vi "System-CAN-Host.vi"() -> ()   [LabVIEW 2016]
uses:
  Shared/Typedefs/System-CAN-FrameInfoArray.ctl
  Shared/Typedefs/System-CAN-FrameInfo.ctl
  <vilib>/addons/Software Calibration Management/xSCM/Controls/ID and Element.ctl
  Shared/DSI-Shared.lvlib
  <vilib>/addons/Software Calibration Management/xSCM/SCM-API.lvlib
panel:
  in  "QueueLength":u8 caption="Queue Length"
  in  "WritePeriod":u32 caption="[msec]"
  in  "Interface":u8(ring) items=["CAN 0", "CAN 1"]
  in  "BaudRate":u32 caption="[baud]"
  in  "Reset":bool
  out "WriteError":bool
  out "ReadError":bool
  in  "_WriteTable":i32(listbox) caption="Write to CAN Bus"
  in  "_ReadTable":i32(listbox) caption="Read from CAN Bus"
  in  "_Hidden":enum32{"Page 1"}(tab)
  in  "_Edit":bool
  in  "_Down":bool
  in  "_Delete":bool
  in  "_Up":bool
  in  "_Insert":bool
  out "ReadElements":i32
  out "WriteElements":i32
  in  "_Read(F)-Write(T)":bool
  in  "_Refresh":bool
  out "Read_ActIDs":sgl[](array[numeric])
  out "Read_Values":sgl[](array[numeric])
  out "Write_Values":sgl[](array[numeric])
  in  "Read_IDs":sgl[](array[numeric])
  in  "ReadFramesInfo":T1
  in  "WriteFramesInfo":T1
  in  "_CurrentFrameInfo":T2
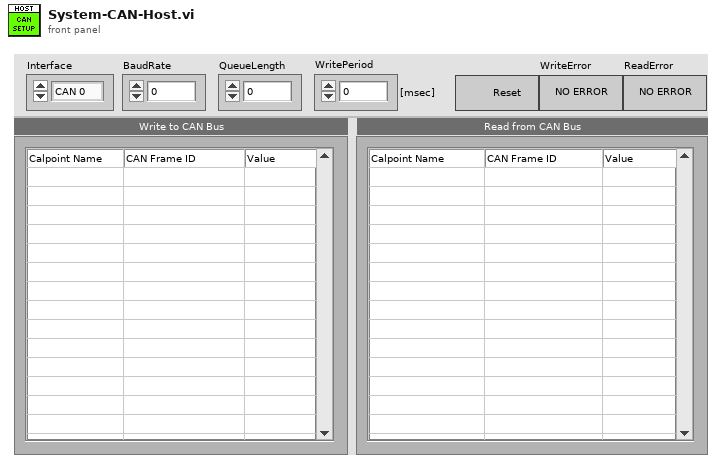
[diagram p1: front panel]
types:
  T1 = typedef "DSI-Shared.lvlib/System-CAN-FrameInfoArray.ctl" = T2[]
  T2 = typedef "DSI-Shared.lvlib/System-CAN-FrameInfo.ctl" = cluster{"Name":string, "Units":string, "Identifier":u32, "Disable":bool, "Type":u16, "Scaling Factor":sgl, "Offset":sgl, "ExtID":bool, "Min":sgl, "Max":sgl, "Number of Bits":u8, "Start Bit":u8, "Byte Order":u8, "ID":T3}
  T3 = typedef "SCM-API.lvlib/ID and Element.ctl" = cluster{"ID":u32, "Element":i32[]}
  T4 = typedef "LVBoundsTypeDef.ctl" = cluster{"Width":u32, "Height":u32}
  T5 = typedef "LVRectTypeDef.ctl" = cluster{"Left":i16, "Top":i16, "Right":i16, "Bottom":i16}
  T6 = typedef "LVRowAndColumnUnsignedTypeDef.ctl" = cluster{"Row":u32, "Column":u32}
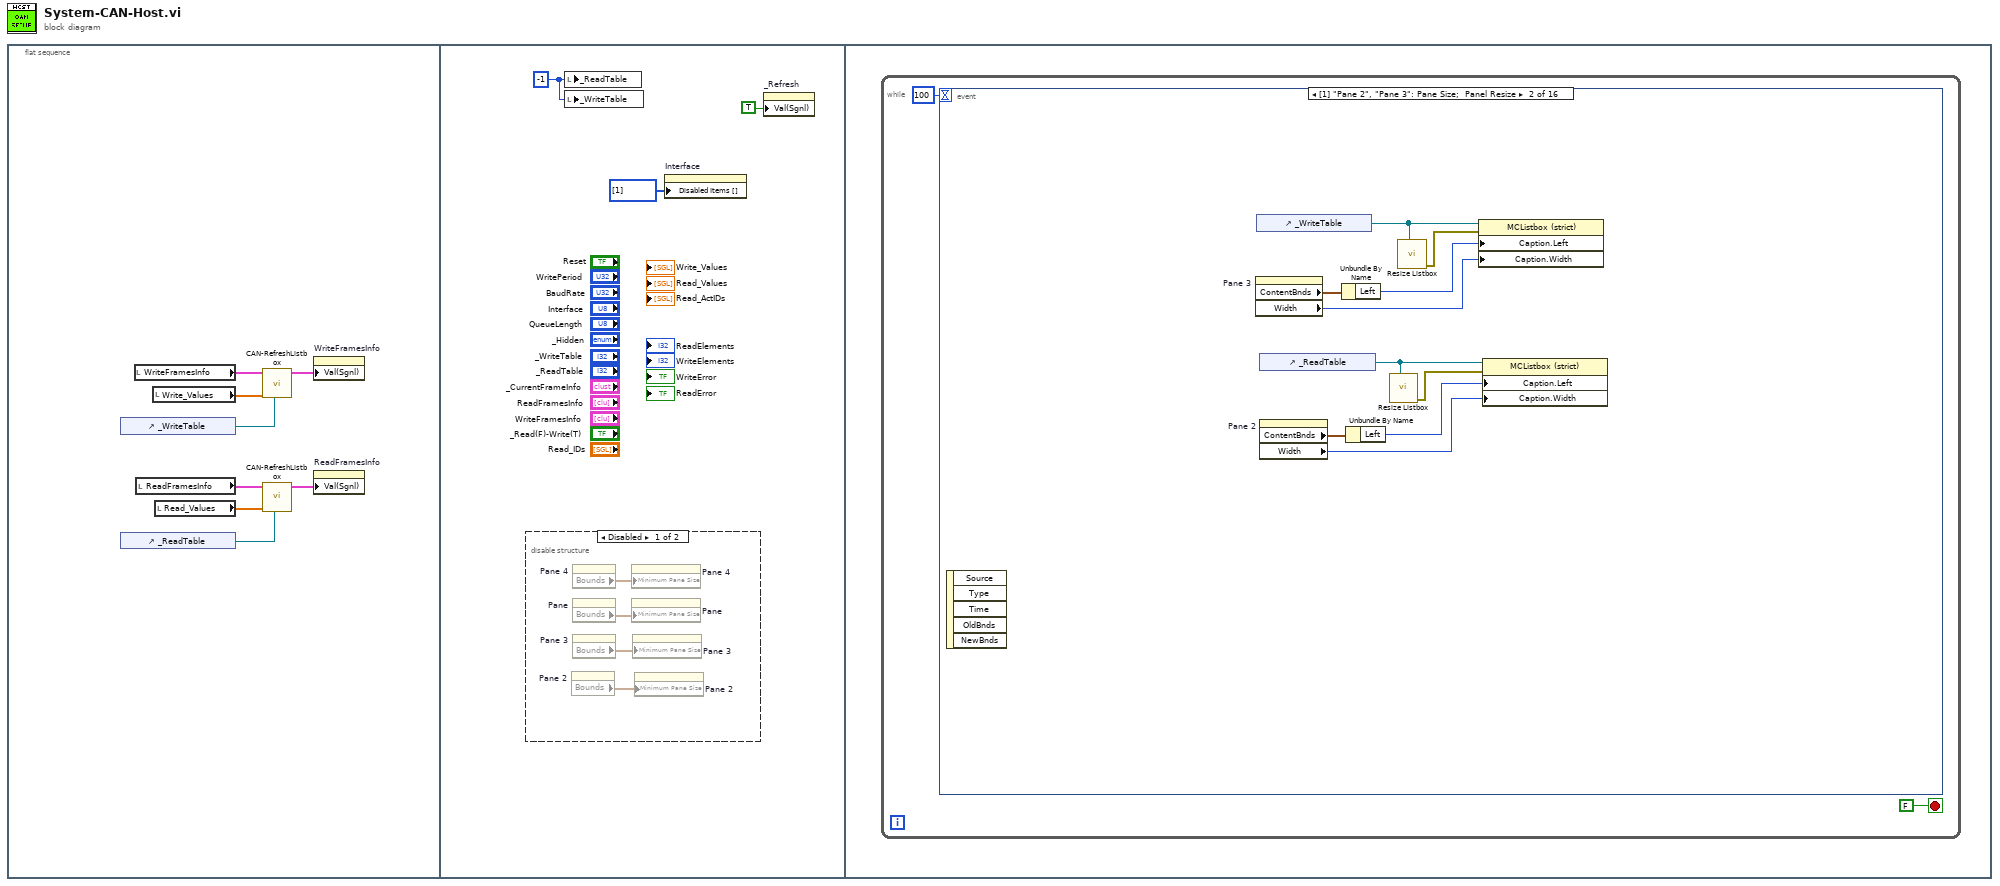
[diagram p0: block diagram]
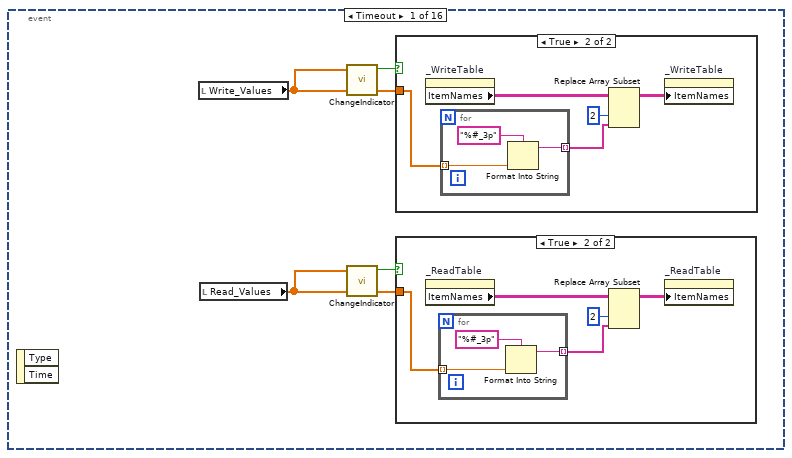
[diagram p3: hidden frame]
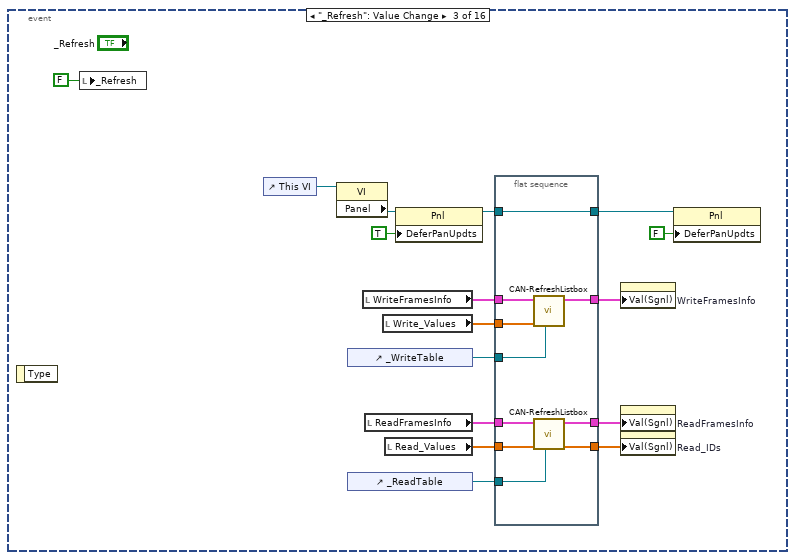
[diagram p6: hidden frame]
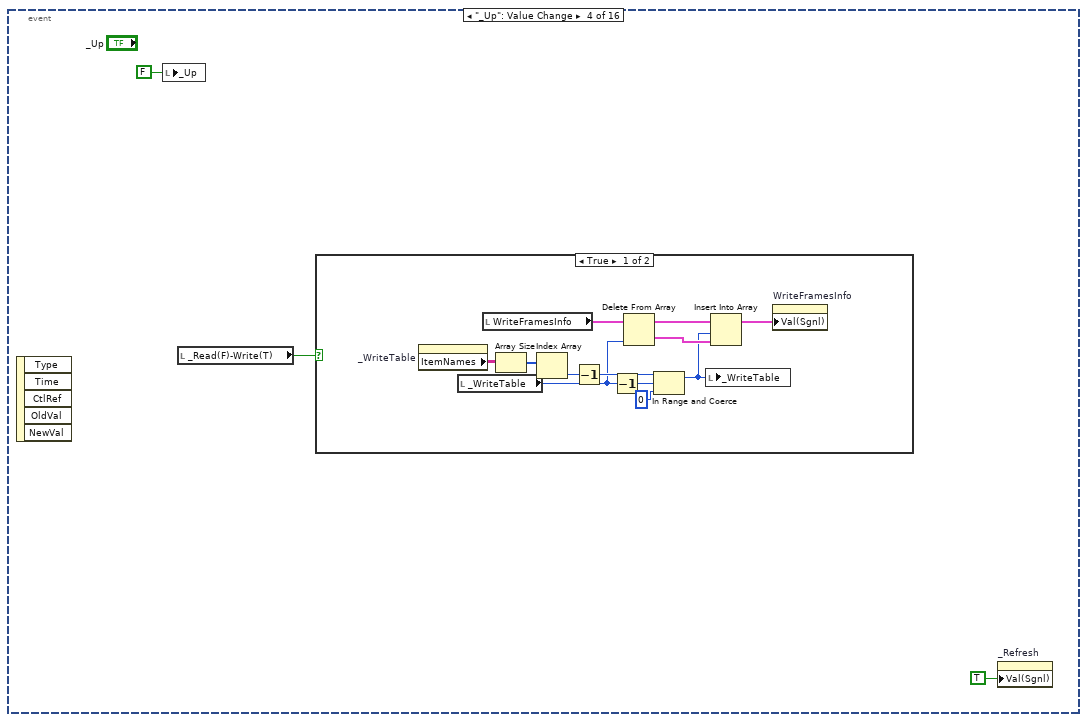
[diagram p7: hidden frame]
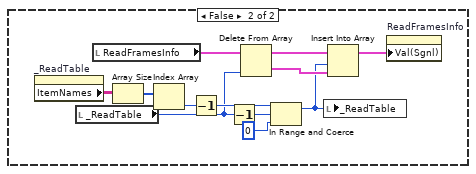
[diagram p8: hidden frame]
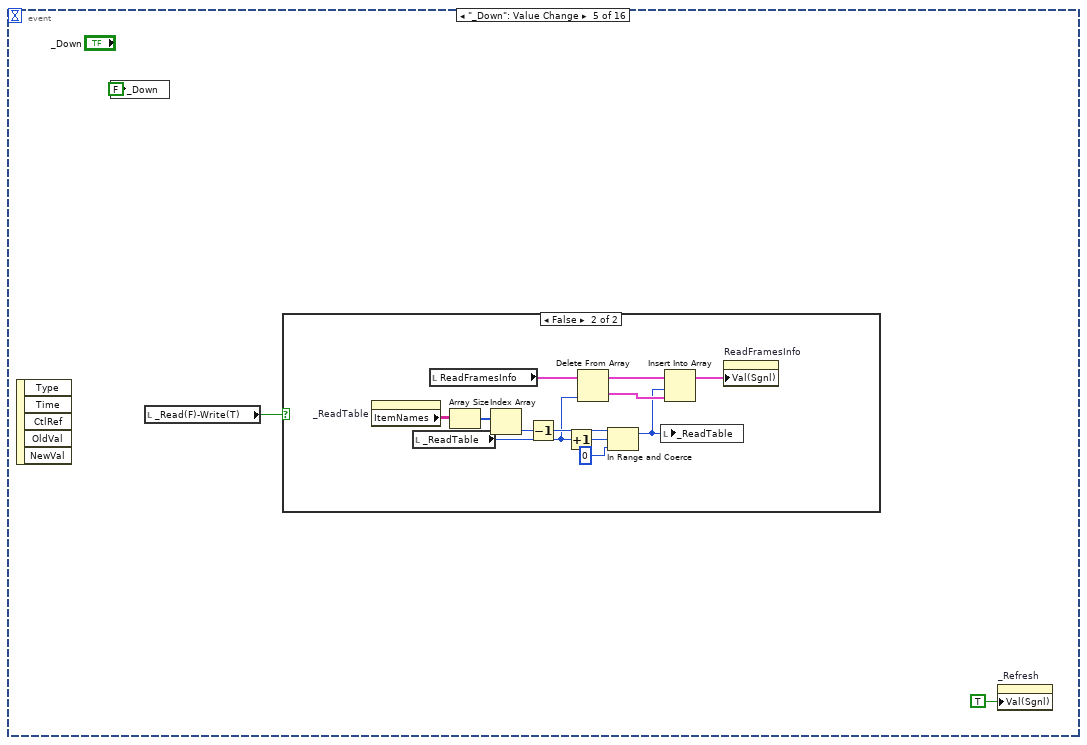
[diagram p9: hidden frame]
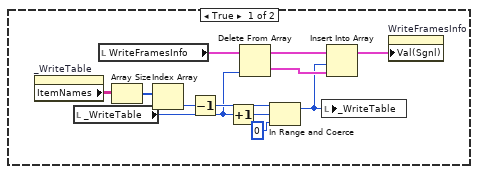
[diagram p10: hidden frame]
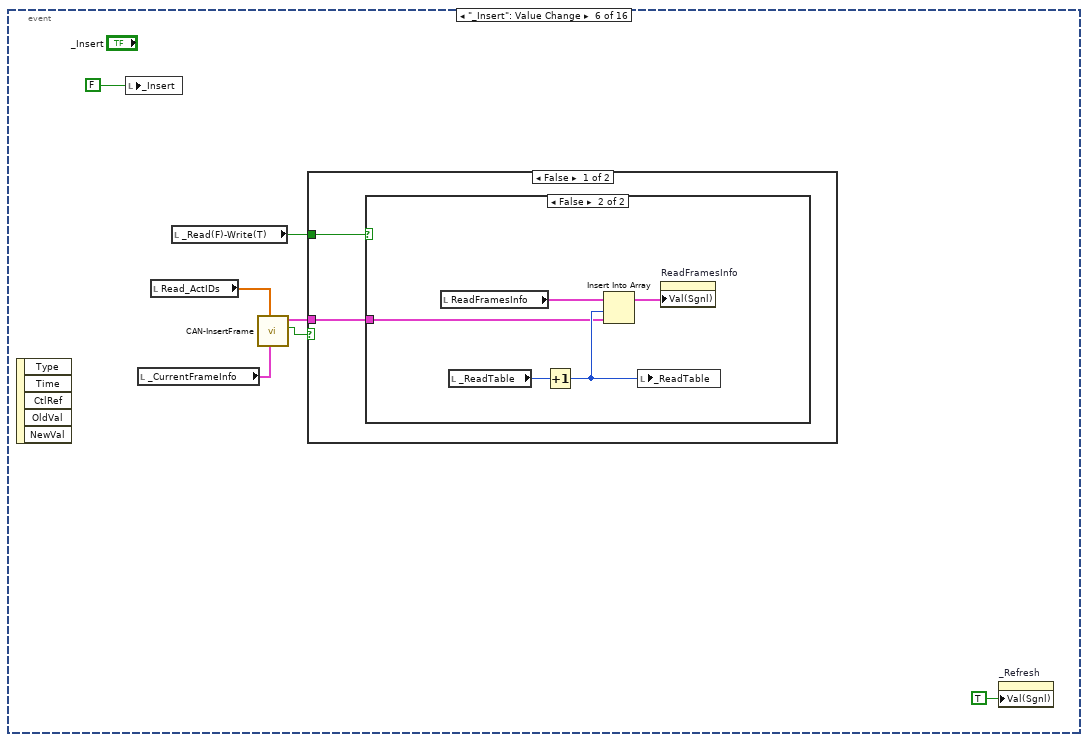
[diagram p11: hidden frame]
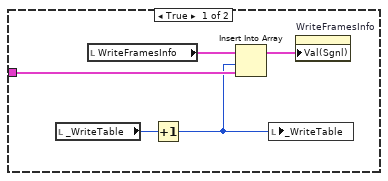
[diagram p12: hidden frame]
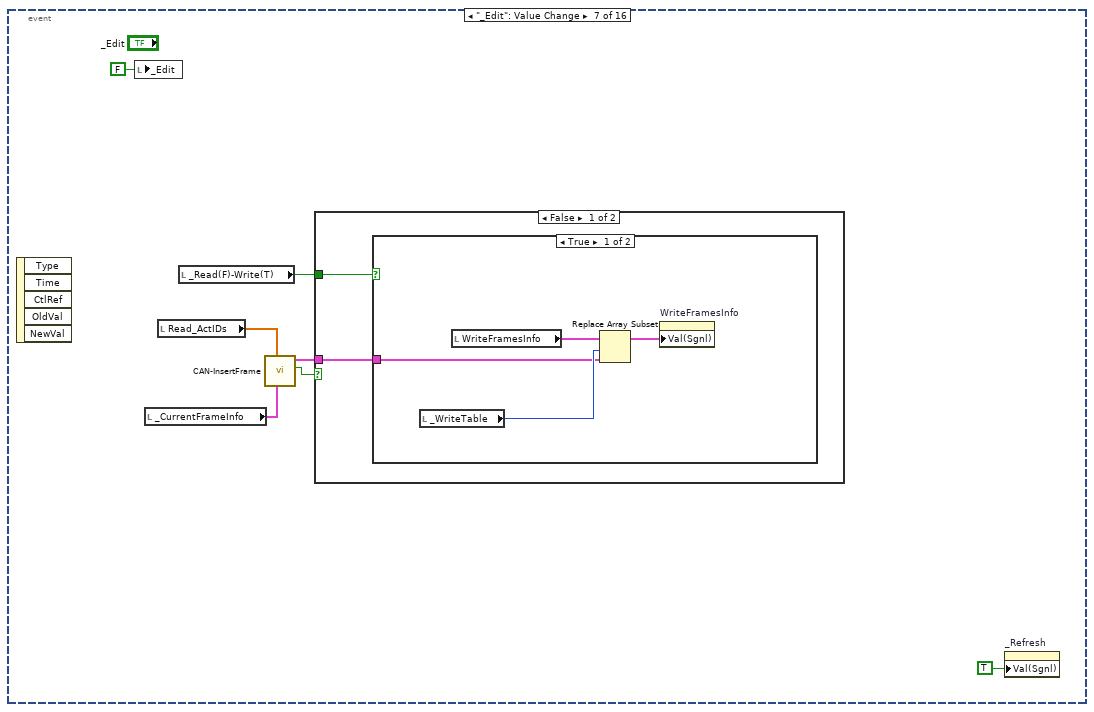
[diagram p14: hidden frame]
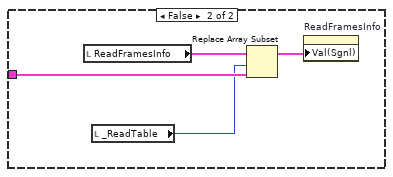
[diagram p15: hidden frame]
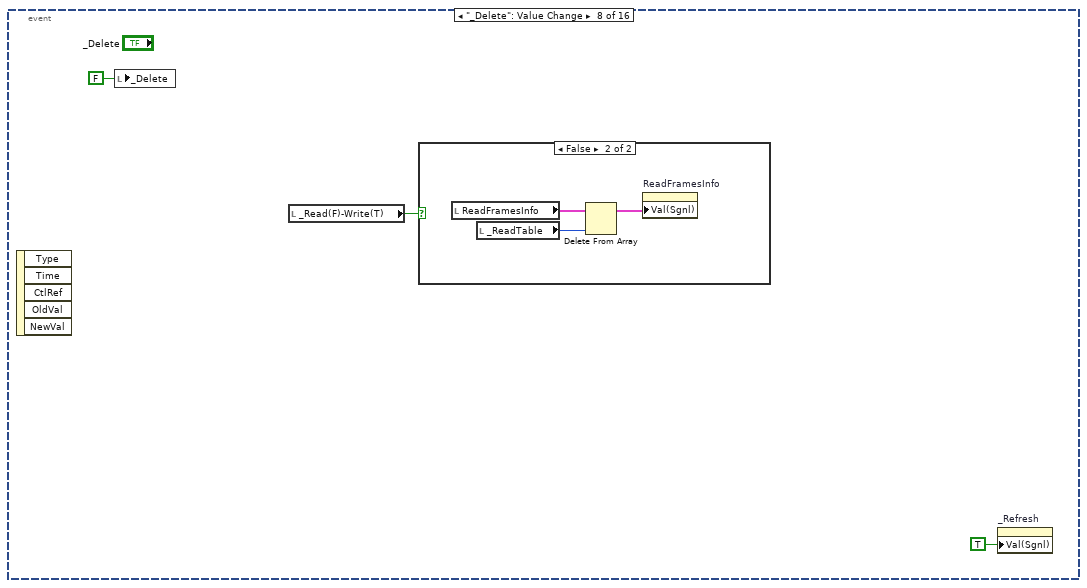
[diagram p17: hidden frame]
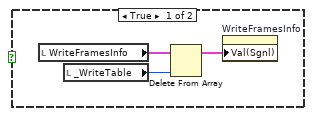
[diagram p18: hidden frame]
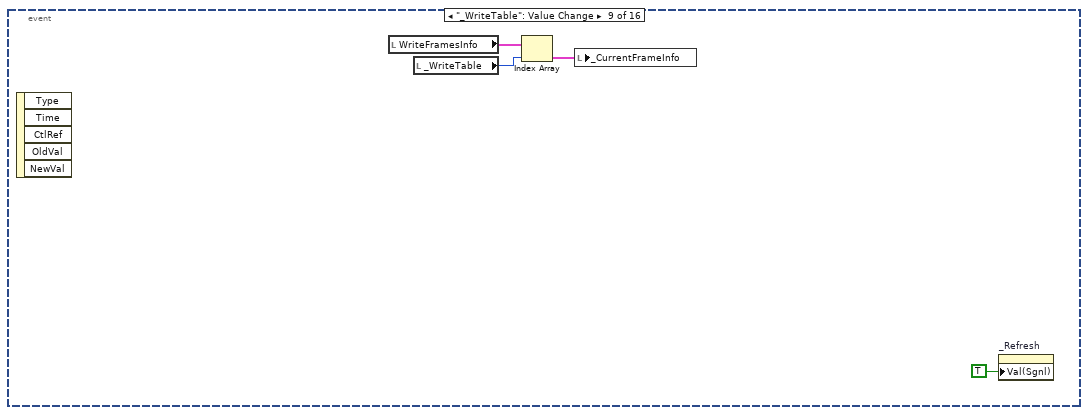
[diagram p19: hidden frame]
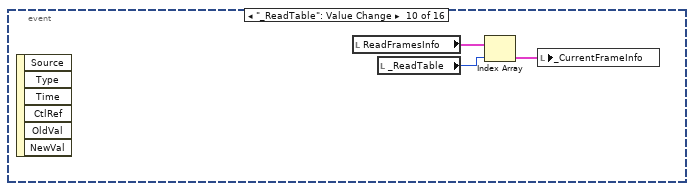
[diagram p20: hidden frame]
diagram:
  n1 = flat-sequence {
    frame #0 {
      n2 = control-ref of="_WriteTable"() -> (w6:refnum<vi>)
      n3 = control-ref of="_ReadTable"() -> (w5:refnum<vi>)
      n4 = local read "WriteFramesInfo"() -> (w8:T1)
      n5 = local read "ReadFramesInfo"() -> (w3:T1)
      n6 = local read "Write_Values"() -> (w7:sgl[])
      n7 = local read "Read_Values"() -> (w4:sgl[])
      n8 = call "CAN-RefreshListbox.vi"("Table"=w6, "Values"=w7, "FramesInfo"=w8) -> ("FramesInfo"=w1:T1)  [unwired: 7 in, 1 out]
      n9 = call "CAN-RefreshListbox.vi"("Table"=w5, "Values"=w4, "FramesInfo"=w3) -> ("FramesInfo"=w2:T1)  [unwired: 7 in, 1 out]
      n10 = property on="WriteFramesInfo" class="Arr (strict)"("Val(Sgnl)"=w1) -> ()  [unwired: 2 in, 2 out]
      n11 = property on="ReadFramesInfo" class="Arr (strict)"("Val(Sgnl)"=w2) -> ()  [unwired: 2 in, 2 out]
    }
    frame #1 {
      w10 = -1 ("_ReadTable")
      n12 = disable-structure shown="Disabled" {
        frame Disabled {
          n13 = property on="Pane 2" class="Pane"() -> ("Bounds"=w12:T4)  [unwired: 2 in, 2 out]
          n14 = property on="Pane 4" class="Pane"() -> ("Bounds"=w15:T4)  [unwired: 2 in, 2 out]
          n15 = property on="Pane" class="Pane"() -> ("Bounds"=w14:T4)  [unwired: 2 in, 2 out]
          n16 = property on="Pane 3" class="Pane"() -> ("Bounds"=w13:T4)  [unwired: 2 in, 2 out]
          n17 = property on="Pane 4" class="Pane"("Minimum Pane Size"=w15) -> ()  [unwired: 2 in, 2 out]
          n18 = property on="Pane" class="Pane"("Minimum Pane Size"=w14) -> ()  [unwired: 2 in, 2 out]
          n19 = property on="Pane 3" class="Pane"("Minimum Pane Size"=w13) -> ()  [unwired: 2 in, 2 out]
          n20 = property on="Pane 2" class="Pane"("Minimum Pane Size"=w12) -> ()  [unwired: 2 in, 2 out]
        }
        frame Enabled {
        }
      }
      n21 = local write "_ReadTable"(w10) -> ()
      n22 = local write "_WriteTable"(w10) -> ()
      n23 = property on="Interface" class="Ring (strict)"("Disabled Items []"=i32[] [1]) -> ()  [unwired: 2 in, 2 out]
      n24 = property on="_Refresh" class="Bool (strict)"("Val(Sgnl)"=TRUE ("Value (Signaling)")) -> ()  [unwired: 2 in, 2 out]
    }
    frame #2 {
      n25 = while {
        stop <- FALSE stop-if-true
        n26 = event shown="[1] \"Pane 2\", \"Pane 3\": Pane Size;  Panel Resize" {
          selector: _ -> [_ _ _ _ _ _ _ _ _ _ _ _ _ _ _ _]
          dyn-events: _ -> [_ _ _ _ _ _ _ _ _ _ _ _ _ _ _ _]
          timeout: 100 -> [_ _ _ _ _ _ _ _ _ _ _ _ _ _ _ _]
          event Timeout {
            n27 = event-data() -> ()  [unwired: 1 in, 2 out]
            n28 = local read "Write_Values"() -> (w20:sgl[])
            n29 = local read "Read_Values"() -> (w19:sgl[])
            n30 = call "ChangeIndicator.vi"("Input"=w20) -> ("Change"=w21:bool)  [unwired: 9 in]
            n31 = call "ChangeIndicator.vi"("Input"=w19) -> ("Change"=w18:bool)  [unwired: 9 in]
            n32 = case shown="True" w21 {
              tunnel: w20 -> [_ w31]
              frame False {
              }
              frame True {
                n33 = property on="_WriteTable" class="MCListbox (strict)"() -> ("ItemNames"=w34:string[][])  [unwired: 2 in, 2 out]
                n34 = for {
                  tunnel: w31 -> [w37] mode=indexing
                  tunnel: [w35] -> w30 mode=indexing
                  n35 = Format Into String(format string="%#_3p", w37) -> (resulting string=w35:string)  [unwired: 2 in, 1 out]
                }
                n36 = Replace Array Subset(array=w34, new element=w30, index (col)=2 ("disabled index (col)")) -> (w33:string[][])  [unwired: 1 in]
                n37 = property on="_WriteTable" class="MCListbox (strict)"("ItemNames"=w33) -> ()  [unwired: 2 in, 2 out]
              }
            }
            n38 = case shown="True" w18 {
              tunnel: w19 -> [_ w23]
              frame False {
              }
              frame True {
                n39 = property on="_ReadTable" class="MCListbox (strict)"() -> ("ItemNames"=w25:string[][])  [unwired: 2 in, 2 out]
                n40 = for {
                  tunnel: w23 -> [w29] mode=indexing
                  tunnel: [w27] -> w22 mode=indexing
                  n41 = Format Into String(format string="%#_3p", w29) -> (resulting string=w27:string)  [unwired: 2 in, 1 out]
                }
                n42 = Replace Array Subset(array=w25, new element=w22, index (col)=2 ("disabled index (col)")) -> (w24:string[][])  [unwired: 1 in]
                n43 = property on="_ReadTable" class="MCListbox (strict)"("ItemNames"=w24) -> ()  [unwired: 2 in, 2 out]
              }
            }
          }
          event Pane Size; Panel Resize {
            n44 = event-data() -> ()  [unwired: 1 in, 5 out]
            n45 = property on="Pane 3" class="Pane"() -> ("ContentBnds"=w47:T5, "Width"=w45:u32)  [unwired: 2 in, 2 out]
            n46 = control-ref of="_WriteTable"() -> (w38:refnum<vi>)
            n47 = control-ref of="_ReadTable"() -> (w41:refnum<vi>)
            n48 = property on="Pane 2" class="Pane"() -> ("ContentBnds"=w44:T5, "Width"=w42:u32)  [unwired: 2 in, 2 out]
            n49 = Unbundle By Name(w47) -> ("Left"=w46:i16)
            n50 = Unbundle By Name(w44) -> ("Left"=w43:i16)
            n51 = call "Resize Listbox.vi"("MulticolumnListbox in"=w41) -> ("error out"=w40:errorcluster)  [unwired: 10 in]
            n52 = call "Resize Listbox.vi"("MulticolumnListbox in"=w38) -> ("error out"=w39:errorcluster)  [unwired: 10 in]
            n53 = property on="Property Node" class="MCListbox (strict)"(reference=w38, error in=w39, "Caption.Left"=w46, "Caption.Width"=w45) -> ()  [unwired: 2 out]
            n54 = property on="Property Node" class="MCListbox (strict)"(reference=w41, error in=w40, "Caption.Left"=w43, "Caption.Width"=w42) -> ()  [unwired: 2 out]
          }
          event "_Refresh": Value Change {
            n55 = event-data() -> ()  [unwired: 1 in, 1 out]
            n56 = local write "_Refresh"(FALSE ("_Refresh")) -> ()
            n57 = control-ref of="This VI"() -> (w61:refnum<vi>)
            n58 = property class="VI"(reference=w61) -> ("Panel"=w60:refnum<vi>)  [unwired: 1 in, 2 out]
            n59 = control-ref of="_WriteTable"() -> (w62:refnum<vi>)
            n60 = control-ref of="_ReadTable"() -> (w55:refnum<vi>)
            n61 = local read "WriteFramesInfo"() -> (w54:T1)
            n62 = local read "ReadFramesInfo"() -> (w53:T1)
            n63 = local read "Write_Values"() -> (w51:sgl[])
            n64 = local read "Read_Values"() -> (w52:sgl[])
            n65 = property class="Pnl"(reference=w60, "DeferPanUpdts"=TRUE ("Defer Panel Updates")) -> (reference out=w57:refnum<vi>)  [unwired: 1 in, 1 out]
            n66 = flat-sequence {
              tunnel: w62 -> [w72]
              tunnel: w57 -> [w73]
              tunnel: [w73] -> w56
              tunnel: w55 -> [w71]
              tunnel: w54 -> [w70]
              tunnel: w53 -> [w69]
              tunnel: w52 -> [w68]
              tunnel: w51 -> [w67]
              tunnel: [w66] -> w50
              tunnel: [w65] -> w49
              tunnel: [w64] -> w48
              frame #0 {
                n67 = call "CAN-RefreshListbox.vi"("Table"=w72, "Values"=w67, "FramesInfo"=w70) -> ("FramesInfo"=w66:T1)  [unwired: 7 in, 1 out]
                n68 = call "CAN-RefreshListbox.vi"("Table"=w71, "Values"=w68, "FramesInfo"=w69) -> ("IDs"=w64:sgl[], "FramesInfo"=w65:T1)  [unwired: 7 in]
              }
            }
            n69 = property on="WriteFramesInfo" class="Arr (strict)"("Val(Sgnl)"=w50) -> ()  [unwired: 2 in, 2 out]
            n70 = property on="ReadFramesInfo" class="Arr (strict)"("Val(Sgnl)"=w49) -> ()  [unwired: 2 in, 2 out]
            n71 = property on="Read_IDs" class="Arr (strict)"("Val(Sgnl)"=w48) -> ()  [unwired: 2 in, 2 out]
            n72 = property class="Pnl"(reference=w56, "DeferPanUpdts"=FALSE ("Defer Panel Updates")) -> ()  [unwired: 1 in, 2 out]
          }
          event "_Up": Value Change {
            n73 = event-data() -> ()  [unwired: 1 in, 5 out]
            n74 = local write "_Up"(FALSE ("_Up")) -> ()
            n75 = local read "_Read(F)-Write(T)"() -> (w74:bool)
            n76 = case shown="True" w74 {
              frame True {
                n77 = property on="_WriteTable" class="MCListbox (strict)"() -> ("ItemNames"=w83:string[][])  [unwired: 2 in, 2 out]
                n78 = local read "_WriteTable"() -> (w78:i32)
                n79 = local read "WriteFramesInfo"() -> (w82:T1)
                n80 = Array Size(array=w83) -> (size(s)=w85:i32[])
                n81 = Index Array(array=w85) -> (element=w84:i32)  [unwired: 1 in]
                n82 = Decrement(x=w84) -> (x-1=w87:i32)
                n83 = Decrement(x=w78) -> (x-1=w86:i32)
                n84 = Delete From Array(array=w82, index=w78) -> (deleted portion=w80:T2, array with subset deleted=w81:T1)  [unwired: 1 in]
                n85 = In Range and Coerce(upper limit=w87, x=w86, lower limit=0) -> (coerced(x)=w79:i32)  [unwired: 1 out]
                n86 = local write "_WriteTable"(w79) -> ()
                n87 = Insert Into Array(array=w81, index=w79, new element=w80) -> (w77:T1)
                n88 = property on="WriteFramesInfo" class="Arr (strict)"("Val(Sgnl)"=w77) -> ()  [unwired: 2 in, 2 out]
              }
              frame False {
                n89 = property on="_ReadTable" class="MCListbox (strict)"() -> ("ItemNames"=w90:string[][])  [unwired: 2 in, 2 out]
                n90 = local read "_ReadTable"() -> (w92:i32)
                n91 = local read "ReadFramesInfo"() -> (w91:T1)
                n92 = Array Size(array=w90) -> (size(s)=w97:i32[])
                n93 = Index Array(array=w97) -> (element=w96:i32)  [unwired: 1 in]
                n94 = Decrement(x=w96) -> (x-1=w99:i32)
                n95 = Decrement(x=w92) -> (x-1=w98:i32)
                n96 = Delete From Array(array=w91, index=w92) -> (deleted portion=w94:T2, array with subset deleted=w95:T1)  [unwired: 1 in]
                n97 = In Range and Coerce(upper limit=w99, x=w98, lower limit=0) -> (coerced(x)=w93:i32)  [unwired: 1 out]
                n98 = local write "_ReadTable"(w93) -> ()
                n99 = Insert Into Array(array=w95, index=w93, new element=w94) -> (w89:T1)
                n100 = property on="ReadFramesInfo" class="Arr (strict)"("Val(Sgnl)"=w89) -> ()  [unwired: 2 in, 2 out]
              }
            }
            n101 = property on="_Refresh" class="Bool (strict)"("Val(Sgnl)"=TRUE ("Value (Signaling)")) -> ()  [unwired: 2 in, 2 out]
          }
          event "_Down": Value Change {
            n102 = event-data() -> ()  [unwired: 1 in, 5 out]
            n103 = local write "_Down"(FALSE ("_Down")) -> ()
            n104 = local read "_Read(F)-Write(T)"() -> (w101:bool)
            n105 = case shown="False" w101 {
              frame True {
                n106 = property on="_WriteTable" class="MCListbox (strict)"() -> ("ItemNames"=w110:string[][])  [unwired: 2 in, 2 out]
                n107 = local read "_WriteTable"() -> (w105:i32)
                n108 = local read "WriteFramesInfo"() -> (w109:T1)
                n109 = Array Size(array=w110) -> (size(s)=w112:i32[])
                n110 = Index Array(array=w112) -> (element=w111:i32)  [unwired: 1 in]
                n111 = Decrement(x=w111) -> (x-1=w114:i32)
                n112 = Increment(x=w105) -> (x+1=w113:i32)
                n113 = Delete From Array(array=w109, index=w105) -> (deleted portion=w107:T2, array with subset deleted=w108:T1)  [unwired: 1 in]
                n114 = In Range and Coerce(upper limit=w114, x=w113, lower limit=0) -> (coerced(x)=w106:i32)  [unwired: 1 out]
                n115 = local write "_WriteTable"(w106) -> ()
                n116 = Insert Into Array(array=w108, index=w106, new element=w107) -> (w104:T1)
                n117 = property on="WriteFramesInfo" class="Arr (strict)"("Val(Sgnl)"=w104) -> ()  [unwired: 2 in, 2 out]
              }
              frame False {
                n118 = property on="_ReadTable" class="MCListbox (strict)"() -> ("ItemNames"=w117:string[][])  [unwired: 2 in, 2 out]
                n119 = local read "_ReadTable"() -> (w119:i32)
                n120 = local read "ReadFramesInfo"() -> (w118:T1)
                n121 = Array Size(array=w117) -> (size(s)=w124:i32[])
                n122 = Index Array(array=w124) -> (element=w123:i32)  [unwired: 1 in]
                n123 = Decrement(x=w123) -> (x-1=w126:i32)
                n124 = Increment(x=w119) -> (x+1=w125:i32)
                n125 = Delete From Array(array=w118, index=w119) -> (deleted portion=w121:T2, array with subset deleted=w122:T1)  [unwired: 1 in]
                n126 = In Range and Coerce(upper limit=w126, x=w125, lower limit=0) -> (coerced(x)=w120:i32)  [unwired: 1 out]
                n127 = local write "_ReadTable"(w120) -> ()
                n128 = Insert Into Array(array=w122, index=w120, new element=w121) -> (w116:T1)
                n129 = property on="ReadFramesInfo" class="Arr (strict)"("Val(Sgnl)"=w116) -> ()  [unwired: 2 in, 2 out]
              }
            }
            n130 = property on="_Refresh" class="Bool (strict)"("Val(Sgnl)"=TRUE ("Value (Signaling)")) -> ()  [unwired: 2 in, 2 out]
          }
          event "_Insert": Value Change {
            n131 = event-data() -> ()  [unwired: 1 in, 5 out]
            n132 = local write "_Insert"(FALSE ("_Insert")) -> ()
            n133 = local read "_CurrentFrameInfo"() -> (w128:T2)
            n134 = local read "Read_ActIDs"() -> (w130:sgl[])
            n135 = local read "_Read(F)-Write(T)"() -> (w131:bool)
            n136 = call "CAN-InsertFrame.vi"("_FrameInfoIn"=w128, "ActIDs"=w130) -> ("_CANCELED"=w132:bool, "_FrameInfo"=w133:T2)  [unwired: 8 in]
            n137 = case shown="False" w132 {
              tunnel: w133 -> [w135 _]
              tunnel: w131 -> [w136 _]
              frame False {
                n138 = case shown="False" w136 {
                  tunnel: w135 -> [w140 w142]
                  frame True {
                    n139 = local read "_WriteTable"() -> (w141:i32)
                    n140 = local read "WriteFramesInfo"() -> (w137:T1)
                    n141 = Increment(x=w141) -> (x+1=w139:i32)
                    n142 = Insert Into Array(array=w137, index=w139, new element=w140) -> (w138:T1)
                    n143 = local write "_WriteTable"(w139) -> ()
                    n144 = property on="WriteFramesInfo" class="Arr (strict)"("Val(Sgnl)"=w138) -> ()  [unwired: 2 in, 2 out]
                  }
                  frame False {
                    n145 = local read "ReadFramesInfo"() -> (w145:T1)
                    n146 = local read "_ReadTable"() -> (w146:i32)
                    n147 = Increment(x=w146) -> (x+1=w143:i32)
                    n148 = Insert Into Array(array=w145, index=w143, new element=w142) -> (w144:T1)
                    n149 = local write "_ReadTable"(w143) -> ()
                    n150 = property on="ReadFramesInfo" class="Arr (strict)"("Val(Sgnl)"=w144) -> ()  [unwired: 2 in, 2 out]
                  }
                }
              }
              frame True {
              }
            }
            n151 = property on="_Refresh" class="Bool (strict)"("Val(Sgnl)"=TRUE ("Value (Signaling)")) -> ()  [unwired: 2 in, 2 out]
          }
          event "_Edit": Value Change {
            n152 = event-data() -> ()  [unwired: 1 in, 5 out]
            n153 = local write "_Edit"(FALSE ("_Edit")) -> ()
            n154 = local read "_CurrentFrameInfo"() -> (w147:T2)
            n155 = local read "Read_ActIDs"() -> (w148:sgl[])
            n156 = local read "_Read(F)-Write(T)"() -> (w149:bool)
            n157 = call "CAN-InsertFrame.vi"("_FrameInfoIn"=w147, "ActIDs"=w148) -> ("_CANCELED"=w150:bool, "_FrameInfo"=w151:T2)  [unwired: 8 in]
            n158 = case shown="False" w150 {
              tunnel: w151 -> [w154 _]
              tunnel: w149 -> [w155 _]
              frame False {
                n159 = case shown="True" w155 {
                  tunnel: w154 -> [w158 w161]
                  frame True {
                    n160 = local read "_WriteTable"() -> (w159:i32)
                    n161 = local read "WriteFramesInfo"() -> (w156:T1)
                    n162 = Replace Array Subset(array=w156, new element=w158, index=w159) -> (w157:T1)
                    n163 = property on="WriteFramesInfo" class="Arr (strict)"("Val(Sgnl)"=w157) -> ()  [unwired: 2 in, 2 out]
                  }
                  frame False {
                    n164 = local read "ReadFramesInfo"() -> (w163:T1)
                    n165 = local read "_ReadTable"() -> (w160:i32)
                    n166 = Replace Array Subset(array=w163, new element=w161, index=w160) -> (w162:T1)
                    n167 = property on="ReadFramesInfo" class="Arr (strict)"("Val(Sgnl)"=w162) -> ()  [unwired: 2 in, 2 out]
                  }
                }
              }
              frame True {
              }
            }
            n168 = property on="_Refresh" class="Bool (strict)"("Val(Sgnl)"=TRUE ("Value (Signaling)")) -> ()  [unwired: 2 in, 2 out]
          }
          event "_Delete": Value Change {
            n169 = event-data() -> ()  [unwired: 1 in, 5 out]
            n170 = local write "_Delete"(FALSE ("_Delete")) -> ()
            n171 = local read "_Read(F)-Write(T)"() -> (w164:bool)
            n172 = case shown="False" w164 {
              frame True {
                n173 = local read "WriteFramesInfo"() -> (w167:T1)
                n174 = local read "_WriteTable"() -> (w169:i32)
                n175 = Delete From Array(array=w167, index=w169) -> (array with subset deleted=w168:T1)  [unwired: 1 in, 1 out]
                n176 = property on="WriteFramesInfo" class="Arr (strict)"("Val(Sgnl)"=w168) -> ()  [unwired: 2 in, 2 out]
              }
              frame False {
                n177 = local read "ReadFramesInfo"() -> (w171:T1)
                n178 = local read "_ReadTable"() -> (w172:i32)
                n179 = Delete From Array(array=w171, index=w172) -> (array with subset deleted=w170:T1)  [unwired: 1 in, 1 out]
                n180 = property on="ReadFramesInfo" class="Arr (strict)"("Val(Sgnl)"=w170) -> ()  [unwired: 2 in, 2 out]
              }
            }
            n181 = property on="_Refresh" class="Bool (strict)"("Val(Sgnl)"=TRUE ("Value (Signaling)")) -> ()  [unwired: 2 in, 2 out]
          }
          event "_WriteTable": Value Change {
            n182 = event-data() -> ()  [unwired: 1 in, 5 out]
            n183 = local read "WriteFramesInfo"() -> (w174:T1)
            n184 = local read "_WriteTable"() -> (w175:i32)
            n185 = Index Array(array=w174, index=w175) -> (element=w173:T2)
            n186 = local write "_CurrentFrameInfo"(w173) -> ()
            n187 = property on="_Refresh" class="Bool (strict)"("Val(Sgnl)"=TRUE ("Value (Signaling)")) -> ()  [unwired: 2 in, 2 out]
          }
          event "_ReadTable": Value Change {
            n188 = event-data() -> ()  [unwired: 1 in, 6 out]
            n189 = local read "ReadFramesInfo"() -> (w178:T1)
            n190 = local read "_ReadTable"() -> (w179:i32)
            n191 = Index Array(array=w178, index=w179) -> (element=w177:T2)
            n192 = local write "_CurrentFrameInfo"(w177) -> ()
          }
          event "_ReadTable": Mouse Down {
            n193 = event-data() -> ()  [unwired: 1 in, 8 out]
            n194 = local write "_Read(F)-Write(T)"(FALSE ("Read(F)-Write(T)")) -> ()
            n195 = local write "_WriteTable"(-1 ("_WriteTable")) -> ()
          }
          event "_WriteTable": Mouse Down {
            n196 = event-data() -> ()  [unwired: 1 in, 8 out]
            n197 = local write "_Read(F)-Write(T)"(TRUE ("Read(F)-Write(T)")) -> ()
            n198 = local write "_ReadTable"(-1 ("_ReadTable")) -> ()
          }
          event "_WriteTable": Shortcut Menu Activation? {
            w193 = 51  # Header Height
            n199 = event-data() -> ("Coords.Vertical"=w191:i32, "CtlRef"=w192:refnum<vi>, "MenuRef"=w206:refnum<k9>)  [unwired: 1 in]
            n200 = property on="Property Node" class="MCListbox (strict)"(reference=w192) -> ("Top"=w194:i32, "Height"=w196:u32, "TopLeft"=w197:T6, "ItemNames"=w190:string[][])  [unwired: 1 in, 2 out]
            n201 = Delete Menu Items(9:w206) -> (3:w207:refnum<k9>)  [unwired: 3 in, 1 out]
            n202 = Increment(x=w196) -> (x+1=w200:u32)
            n203 = Unbundle By Name(w197) -> ("Row"=w199:u32)
            n204 = Compound Arithmetic op=ADD(invert w193, w191, invert w194) -> (w195:i32)
            n205 = Quotient & Remainder(x=w195, y=w200) -> (floor(x/y)=w198:u32)  [unwired: 1 out]
            n206 = Add(x=w198, y=w199) -> (x+y=w187:u32)
            n207 = Insert Menu Items(7:string[] ["_INSERT", "_EDIT", "_DELETE", "APP_SEPARATOR", "_UP", "_DOWN"], 8:string[] ["Insert", "Edit", "Delete", " ", "Move Up", "Move Down"], 9:w207) -> (3:w203:refnum<k9>)  [unwired: 3 in, 2 out]
            n208 = Index Array(array=w190, index (row)=w187) -> (element=w188:string[])  [unwired: 1 in]
            n209 = Empty String/Path?(string/path=w188) -> (empty?=w186:bool[])
            n210 = And Array Elements(Boolean array=w186) -> (logical AND=w185:bool)
            n211 = Select(t=-1, s=w185, f=w187) -> (s? t:f=w184:u32)
            n212 = for {
              shift-right: [w211] -> _
              shift-left: w203 -> [w212]
              tunnel: string[] ["_EDIT", "_DELETE", "_UP", "_DOWN"] -> [w210] mode=indexing
              tunnel: string[] ["Edit", "Delete", "Move Up", "Move Down"] -> [w209] mode=indexing
              tunnel: w185 -> [w208]
              n213 = Not(x=w208) -> (.not. x?=w213:bool)
              n214 = Set Menu Item Info(7:w210, 9:w213, 10:w209, 11:w212) -> (3:w211:refnum<k9>)  [unwired: 3 in, 1 out]
            }
            n215 = property on="_WriteTable" class="MCListbox (strict)"("Val(Sgnl)"=w184) -> ()  [unwired: 2 in, 2 out]
            n216 = event-data() -> ()  [unwired: 2 in, 1 out]
          }
          event "_ReadTable": Shortcut Menu Activation? {
            w223 = 51  # Header Height
            n217 = event-data() -> ("Coords.Vertical"=w221:i32, "CtlRef"=w222:refnum<vi>, "MenuRef"=w236:refnum<k9>)  [unwired: 1 in]
            n218 = property on="Property Node" class="MCListbox (strict)"(reference=w222) -> ("Top"=w224:i32, "Height"=w226:u32, "TopLeft"=w227:T6, "ItemNames"=w220:string[][])  [unwired: 1 in, 2 out]
            n219 = Delete Menu Items(9:w236) -> (3:w237:refnum<k9>)  [unwired: 3 in, 1 out]
            n220 = Increment(x=w226) -> (x+1=w230:u32)
            n221 = Unbundle By Name(w227) -> ("Row"=w229:u32)
            n222 = Compound Arithmetic op=ADD(invert w223, w221, invert w224) -> (w225:i32)
            n223 = Quotient & Remainder(x=w225, y=w230) -> (floor(x/y)=w228:u32)  [unwired: 1 out]
            n224 = Add(x=w228, y=w229) -> (x+y=w218:u32)
            n225 = Insert Menu Items(7:string[] ["_INSERT", "_EDIT", "_DELETE", "APP_SEPARATOR", "_UP", "_DOWN"], 8:string[] ["Insert", "Edit", "Delete", " ", "Move Up", "Move Down"], 9:w237) -> (3:w233:refnum<k9>)  [unwired: 3 in, 2 out]
            n226 = Index Array(array=w220, index (row)=w218) -> (element=w215:string[])  [unwired: 1 in]
            n227 = Empty String/Path?(string/path=w215) -> (empty?=w216:bool[])
            n228 = And Array Elements(Boolean array=w216) -> (logical AND=w214:bool)
            n229 = Select(t=-1, s=w214, f=w218) -> (s? t:f=w217:u32)
            n230 = for {
              shift-right: [w241] -> _
              shift-left: w233 -> [w242]
              tunnel: string[] ["_EDIT", "_DELETE", "_UP", "_DOWN"] -> [w240] mode=indexing
              tunnel: string[] ["Edit", "Delete", "Move Up", "Move Down"] -> [w239] mode=indexing
              tunnel: w214 -> [w238]
              n231 = Not(x=w238) -> (.not. x?=w243:bool)
              n232 = Set Menu Item Info(7:w240, 9:w243, 10:w239, 11:w242) -> (3:w241:refnum<k9>)  [unwired: 3 in, 1 out]
            }
            n233 = property on="_ReadTable" class="MCListbox (strict)"("Val(Sgnl)"=w217) -> ()  [unwired: 2 in, 2 out]
            n234 = event-data() -> ()  [unwired: 2 in, 1 out]
          }
          event "_WriteTable": Shortcut Menu Selection (User) {
            n235 = event-data() -> ("ItemTag"=w244:string)  [unwired: 1 in]
            n236 = case shown="\"_DELETE\"" w244 {
              frame Default {
              }
              frame "_INSERT" {
                n237 = property on="_Insert" class="Bool (strict)"("Val(Sgnl)"=TRUE ("Value (Signaling)")) -> ()  [unwired: 2 in, 2 out]
              }
              frame "_EDIT" {
                n238 = property on="_Edit" class="Bool (strict)"("Val(Sgnl)"=TRUE ("Value (Signaling)")) -> ()  [unwired: 2 in, 2 out]
              }
              frame "_UP" {
                n239 = property on="_Up" class="Bool (strict)"("Val(Sgnl)"=TRUE ("Value (Signaling)")) -> ()  [unwired: 2 in, 2 out]
              }
              frame "_DOWN" {
                n240 = property on="_Down" class="Bool (strict)"("Val(Sgnl)"=TRUE ("Value (Signaling)")) -> ()  [unwired: 2 in, 2 out]
              }
              frame "_DELETE" {
                n241 = property on="_Delete" class="Bool (strict)"("Val(Sgnl)"=TRUE ("Value (Signaling)")) -> ()  [unwired: 2 in, 2 out]
              }
            }
          }
          event "_ReadTable": Shortcut Menu Selection (User) {
            n242 = event-data() -> ("ItemTag"=w250:string)  [unwired: 1 in]
            n243 = case shown="\"_EDIT\"" w250 {
              frame Default {
              }
              frame "_INSERT" {
                n244 = property on="_Insert" class="Bool (strict)"("Val(Sgnl)"=TRUE ("Value (Signaling)")) -> ()  [unwired: 2 in, 2 out]
              }
              frame "_EDIT" {
                n245 = property on="_Edit" class="Bool (strict)"("Val(Sgnl)"=TRUE ("Value (Signaling)")) -> ()  [unwired: 2 in, 2 out]
              }
              frame "_UP" {
                n246 = property on="_Up" class="Bool (strict)"("Val(Sgnl)"=TRUE ("Value (Signaling)")) -> ()  [unwired: 2 in, 2 out]
              }
              frame "_DOWN" {
                n247 = property on="_Down" class="Bool (strict)"("Val(Sgnl)"=TRUE ("Value (Signaling)")) -> ()  [unwired: 2 in, 2 out]
              }
              frame "_DELETE" {
                n248 = property on="_Delete" class="Bool (strict)"("Val(Sgnl)"=TRUE ("Value (Signaling)")) -> ()  [unwired: 2 in, 2 out]
              }
            }
          }
        }
      }
    }
  }
